vi "PLAN_CREATOR.vi"(8 "error In":errorcluster) -> (0 "error out":errorcluster)   [LabVIEW 2017]
uses:
  <vilib>/Utility/error.llb/DialogType.ctl
  Controls/Ass. Loop Control.ctl
panel:
  in  "PLAN NAME":string(combo)
  in  "CURRENT PLAN TABLE":string[][](table)
  in  "REMOVE PART":bool
  in  "ADD PART":bool
  in  "LIST OF PARTS":string(combo)
  in  "DOORS":string(combo)
  out "USER:-":string
  in  "Stop":bool
  out "DATE/TIME":string
  out "Screen Name":string
  # "Nm"
  # "NOT IN USE"
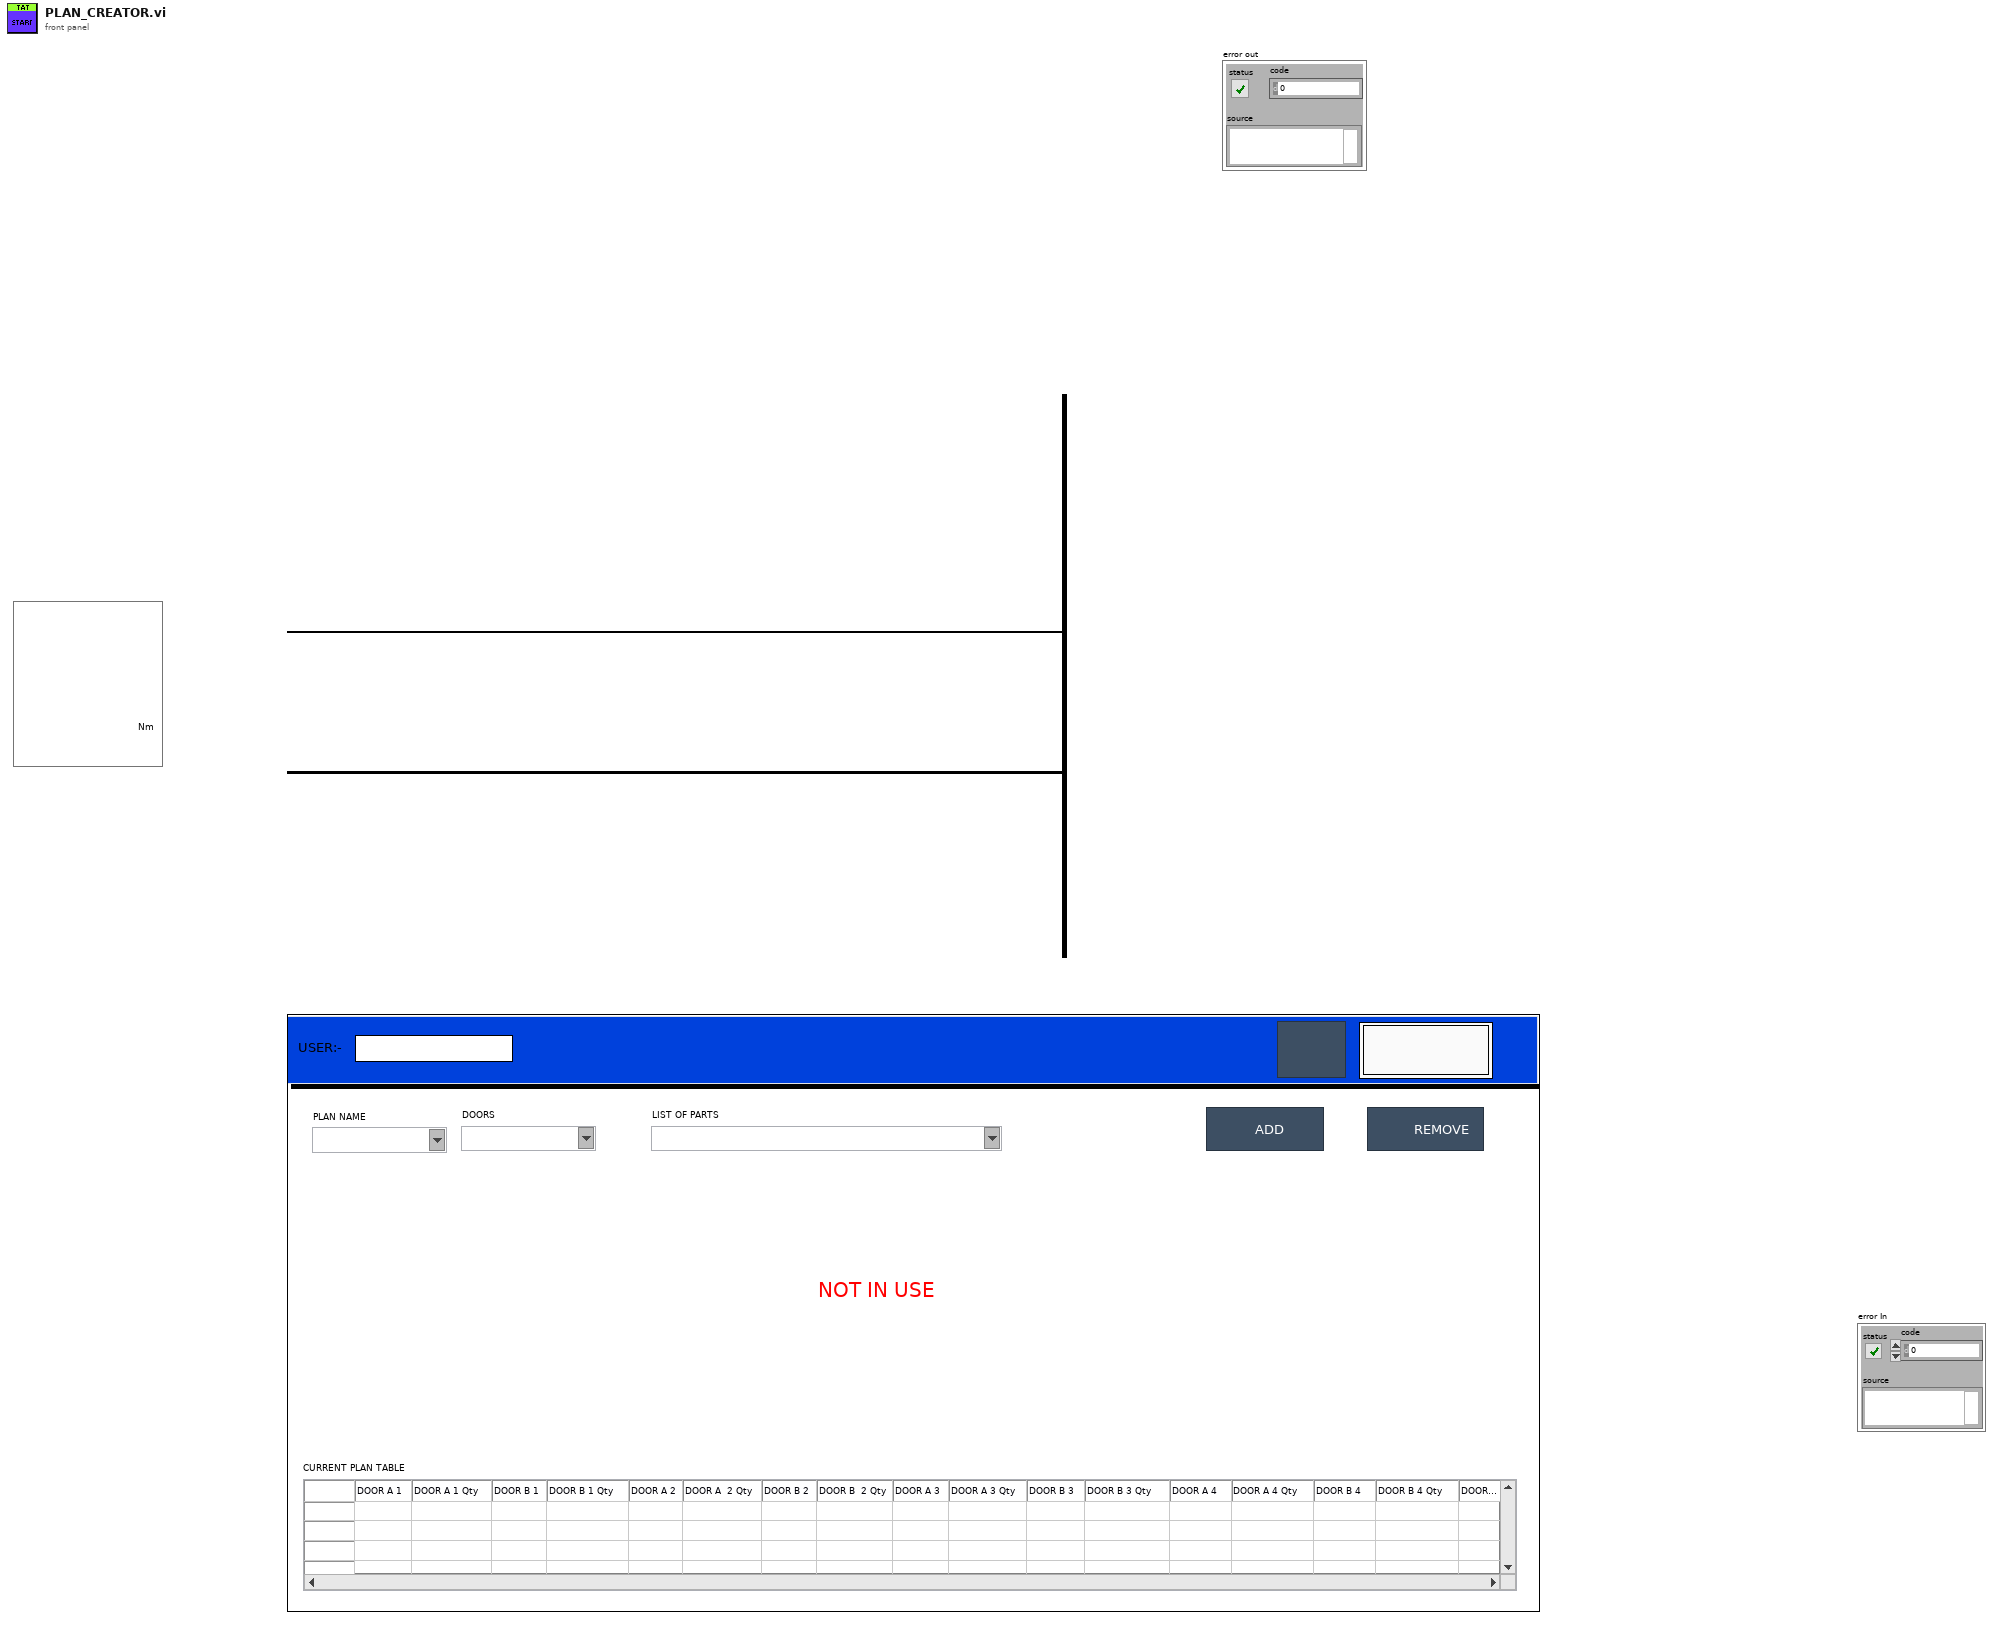
[diagram p1: front panel]
types:
  T1 = typedef "DialogType.ctl" = u16
  T2 = enum32{"invalid app kind", "Development System", "Run Time System", "Student Edition", "Embedded LabVIEW", "Evaluation", "Custom"}
  T3 = typedef "Ass. Loop Control.ctl" = enum16{"Package_Qty_Count", "GENERATE_QR_PRNT", "Cluster_update", "Waiting_for_scan", "barcode CHECK", "Int", "SaveReport ", "Barcode Print", "Start Cycle", "Wait", "Cycle End", "Stop"}
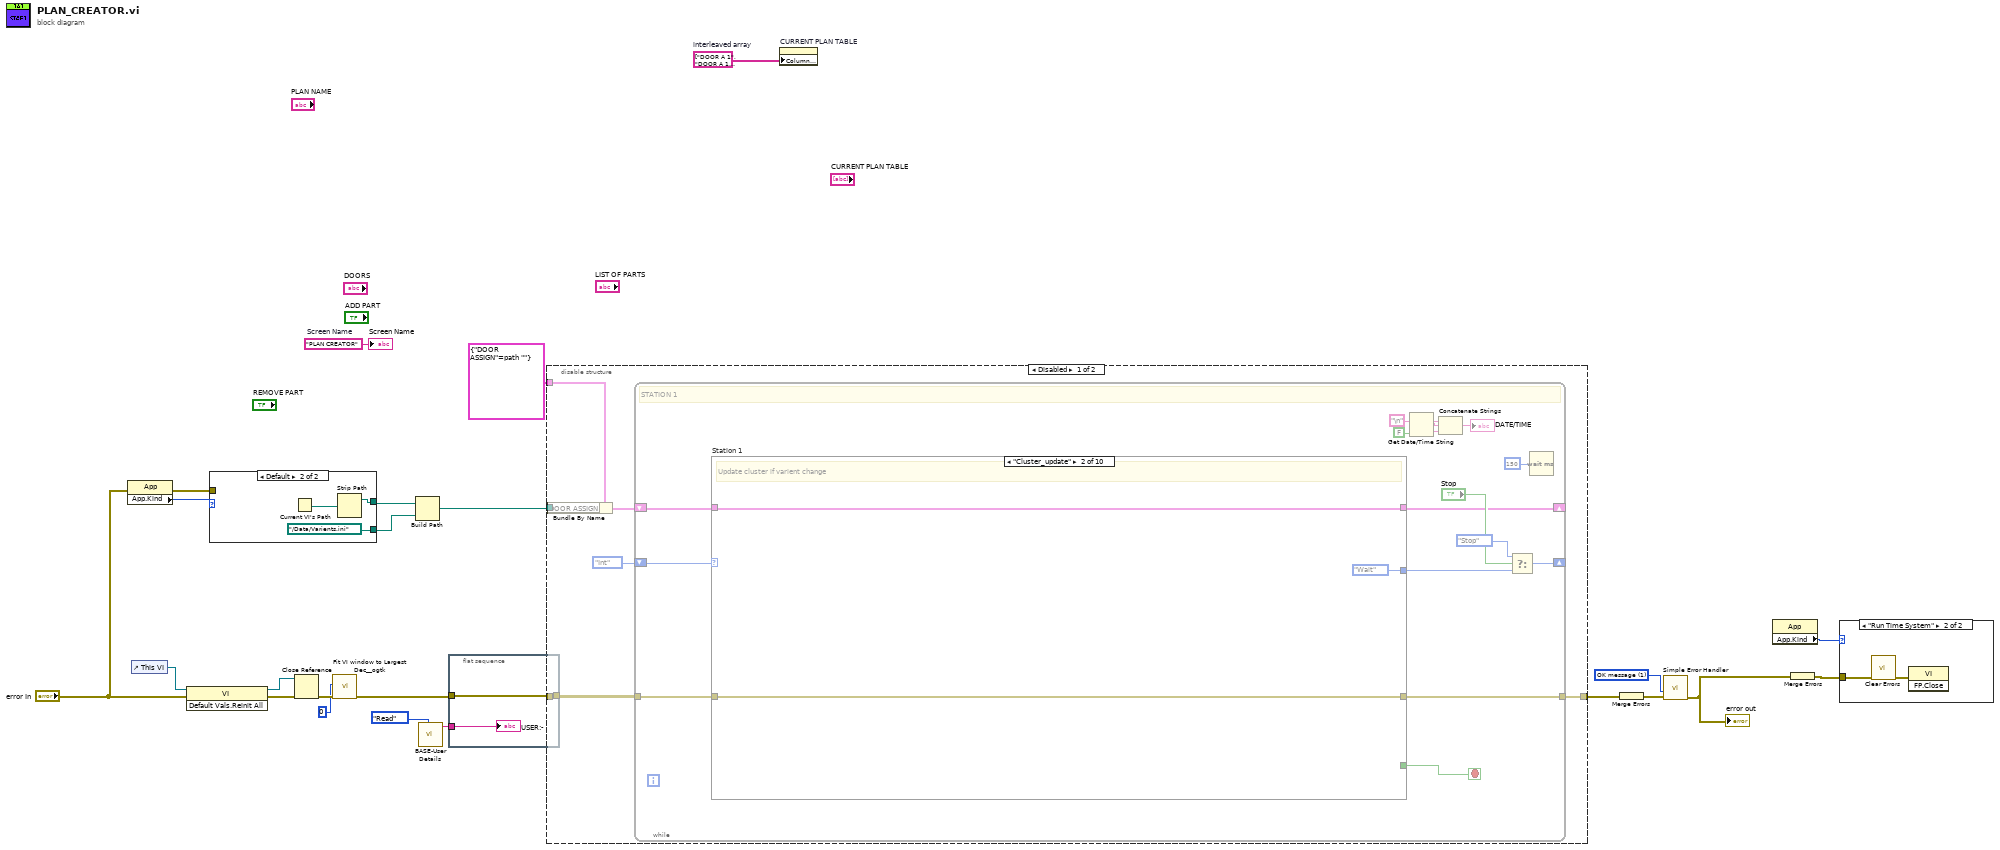
[diagram p0: block diagram]
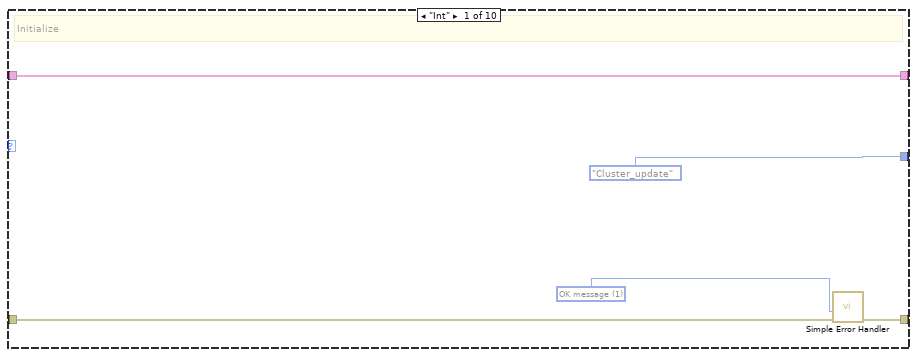
[diagram p2: hidden frame]
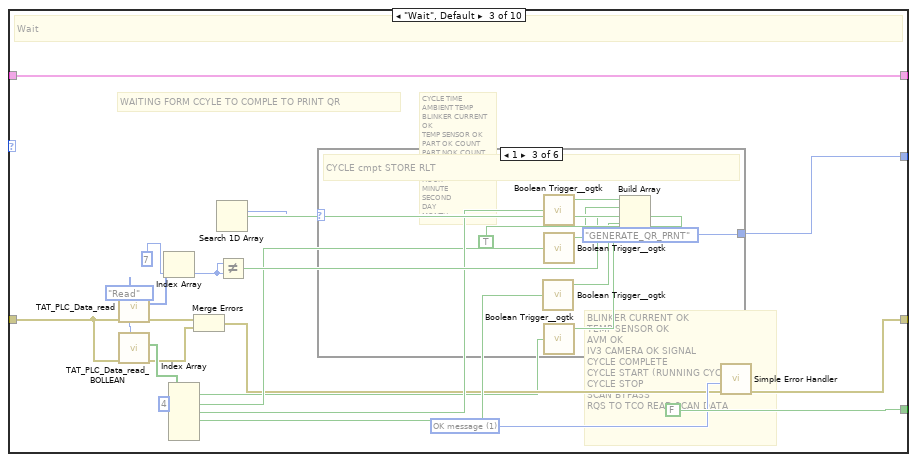
[diagram p3: hidden frame]
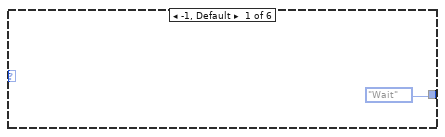
[diagram p4: hidden frame]
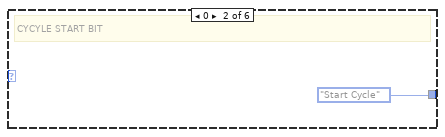
[diagram p5: hidden frame]
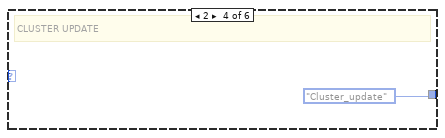
[diagram p6: hidden frame]
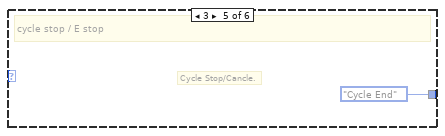
[diagram p7: hidden frame]
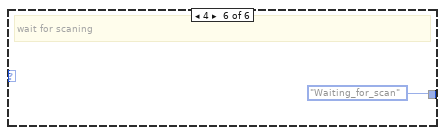
[diagram p8: hidden frame]
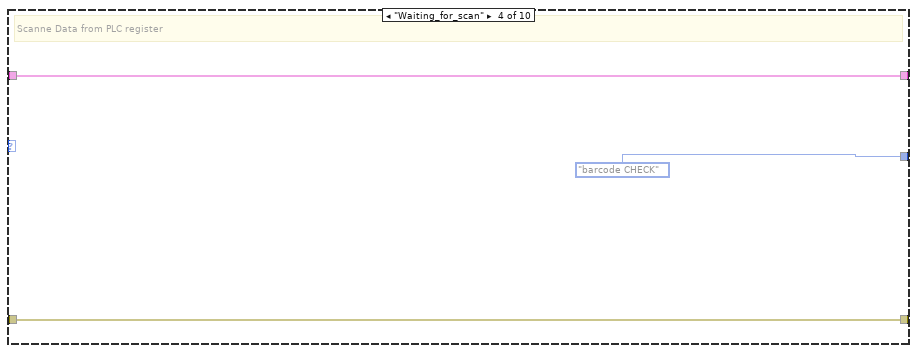
[diagram p9: hidden frame]
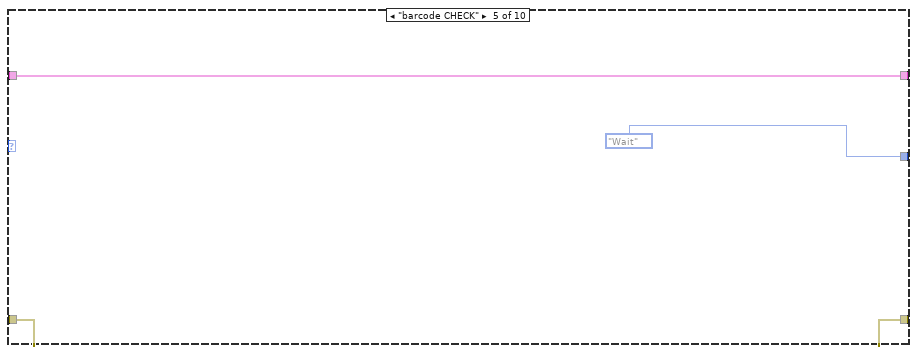
[diagram p10: hidden frame]
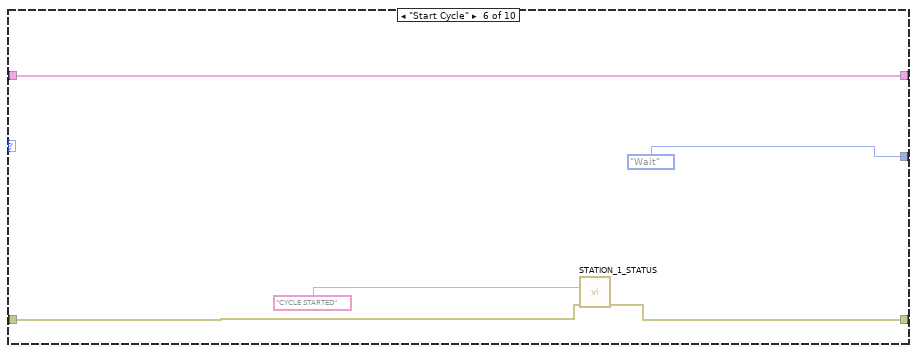
[diagram p11: hidden frame]
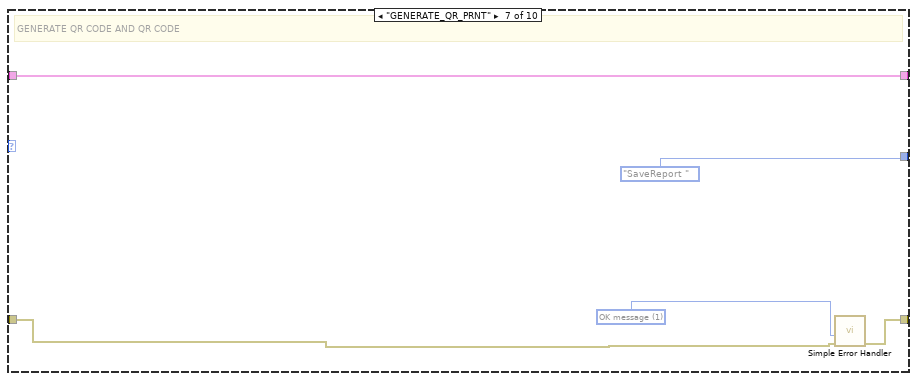
[diagram p12: hidden frame]
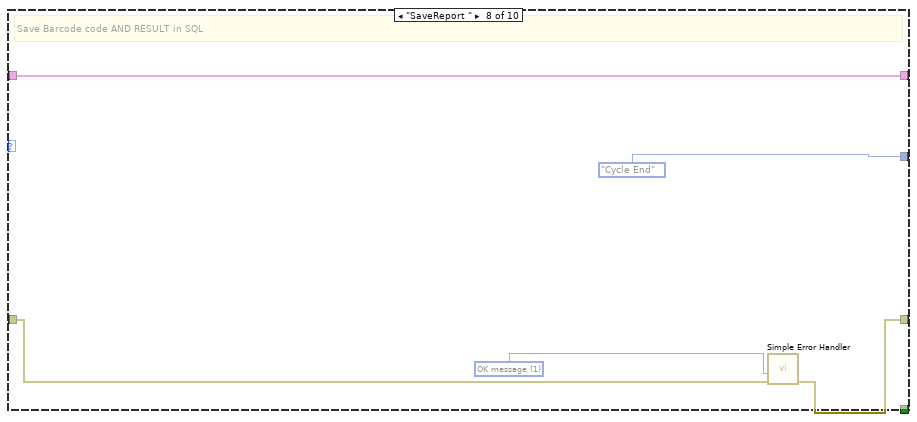
[diagram p13: hidden frame]
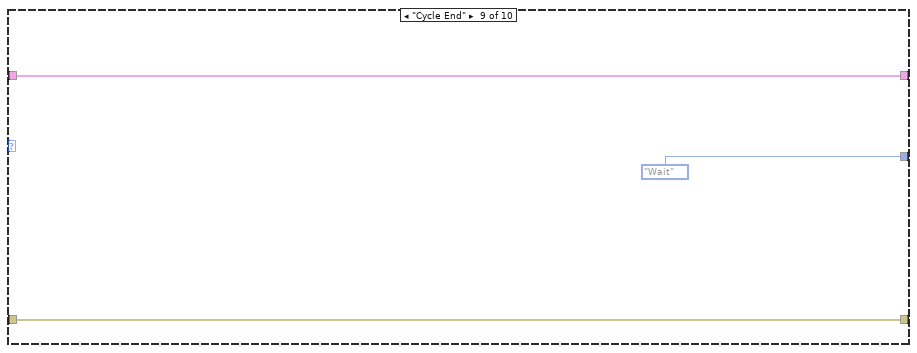
[diagram p14: hidden frame]
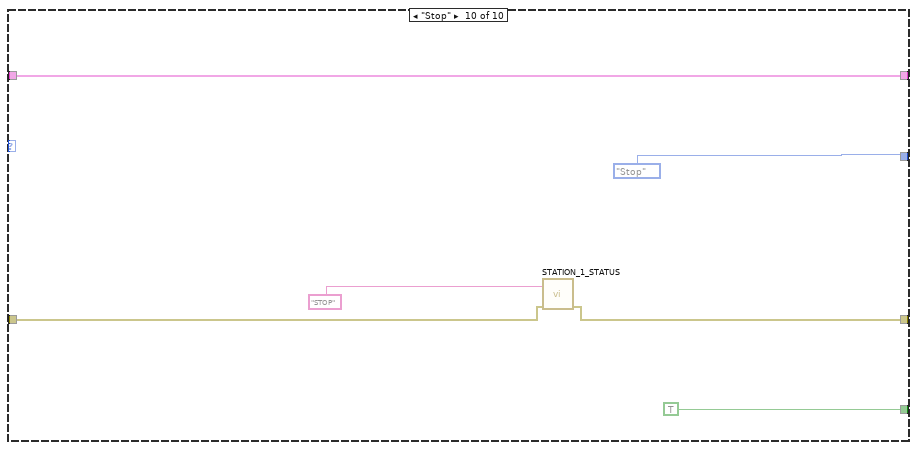
[diagram p15: hidden frame]
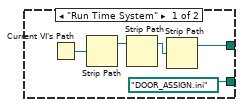
[diagram p17: hidden frame]
diagram:
  w1 = string[] ["DOOR A 1", "DOOR A 1 Qty", "DOOR B 1", "DOOR B 1 Qty", "DOOR A 2", "DOOR A  2 Qty", "DOOR B 2", "DOOR B  2 Qty", "DOOR A 3", "DOOR A 3 Qty", "DOOR B 3", "DOOR B 3 Qty", "DOOR A 4", "DOOR A 4 Qty", "DOOR B 4", "DOOR B 4 Qty", "DOOR A 5", "DOOR A 5 Qty", "DOOR B 5", "DOOR B 5 Qty", "DOOR A 11", "DOOR A 11 Qty", "DOOR B 11", "DOOR B 11 Qty", "DOOR A 12", "DOOR A 12 Qty", "DOOR B 12", "DOOR B 12 Qty", "DOOR A 13", "DOOR A 13 Qty", "DOOR B 13", "DOOR B 13 Qty", "DOOR A 14", "DOOR A 14 Qty", "DOOR B 14", "DOOR B 14 Qty", "DOOR A 15", "DOOR A 15 Qty", "DOOR B 15", "DOOR B 15 Qty", "DOOR A 16", "DOOR A 16 Qty", "DOOR B 16", "DOOR B 16 Qty"]  # interleaved array
  w4 = "PLAN CREATOR"  # Screen Name
  w16 = T1 1 items=["no dialog", "OK message", "continue or stop message", "OK message + warnings", "continue/stop + warnings"] ("type of dialog (OK msg:1)")
  n1 = property class="App"(error in="error In") -> (error out=w12:errorcluster, "App.Kind"=w14:T2)  [unwired: 1 in, 1 out]
  n2 = control-ref of="This VI"() -> (w24:refnum<vi>)
  n3 = invoke class="VI" method="Default Vals.Reinit All"(reference=w24, error in="error In") -> (reference out=w22:refnum<vi>, error out=w23:errorcluster)  [unwired: 1 in, 1 out]
  n4 = case shown="Default" w14 {
    tunnel: [path "DOOR_ASSIGN.ini" ("path") path "../Data/Varients.ini" ("path")] -> w13
    tunnel: [w25 w30] -> w6
    tunnel: w12 -> [_ _]
    frame "Run Time System" {
      n5 = Current VI's Path() -> (path=w28:path)
      n6 = Strip Path(path=w28) -> (stripped path=w27:path)  [unwired: 1 out]
      n7 = Strip Path(path=w27) -> (stripped path=w26:path)  [unwired: 1 out]
      n8 = Strip Path(path=w26) -> (stripped path=w25:path)  [unwired: 1 out]
    }
    frame Default {
      n9 = Current VI's Path() -> (path=w31:path)
      n10 = Strip Path(path=w31) -> (stripped path=w30:path)  [unwired: 1 out]
    }
  }
  n11 = Close Reference(reference=w22, error in (no error)=w23) -> (error out=w21:errorcluster)
  n12 = call <userlib>:"Fit VI window to Largest Dec__ogtk.vi"("error in (no error)"=w21, "border spacing (2 px)"=0) -> ("error out"=w10:errorcluster)  [unwired: 4 in, 1 out]
  n13 = Build Path(base path=w6, name or relative path=w13) -> (appended path=w2:path)
  n14 = call "BASE-User Details.vi"("Enum"=enum16{"Read", "Write"}."Read") -> ("User Name Out"=w17:string)  [unwired: 9 in, 1 out]
  n15 = flat-sequence {
    tunnel: [w34] -> w5
    tunnel: w10 -> [w34]
    tunnel: w17 -> [w33]
    frame #0 {
      "USER:-" <- w33
    }
  }
  n16 = disable-structure shown="Disabled" {
    disable-tunnel: [w39 _] -> w20
    disable-tunnel: w5 -> [w38 _]
    disable-tunnel: cluster{"DOOR ASSIGN":path} {"DOOR ASSIGN"=path ""} -> [w37 _]
    disable-tunnel: w2 -> [w36 _]
    frame Disabled {
      n17 = Bundle By Name(cluster=w37, "DOOR ASSIGN"=w36) -> (w35:cluster{"DOOR ASSIGN":path})
      n18 = while {
        tunnel: w38 -> [w43]
        shift-right: [w53] -> _
        shift-left: Ass._Loop_Control."Int" ("Enum") -> [w56]
        tunnel: [w54] -> w39
        shift-right: [w41] -> _
        shift-left: w35 -> [w42]
        stop <- w46 stop-if-true
        # "STATION 1"
        n19 = case "Station 1" shown="\"Cluster_update\"" w56 {
          tunnel: [Ass._Loop_Control."Cluster_update" ("Enum") Ass._Loop_Control."Wait" ("Enum") w85 Ass._Loop_Control."barcode CHECK" ("Enum") Ass._Loop_Control."Wait" ("Enum") Ass._Loop_Control."Wait" ("Enum") Ass._Loop_Control."SaveReport " ("Enum") Ass._Loop_Control."Cycle End" ("Enum") Ass._Loop_Control."Wait" ("Enum") Ass._Loop_Control."Stop" ("Enum")] -> w45
          tunnel: [_ _ FALSE _ _ _ _ _ _ TRUE] -> w46
          tunnel: [w59 w63 w82 w99 w102 w105 w112 w116 w120 w123] -> w54
          tunnel: w43 -> [w58 w63 w79 w99 w102 w106 w110 w115 w120 w124]
          tunnel: w42 -> [w57 w62 w65 w98 w101 w104 w109 w114 w119 w122]
          tunnel: [w57 w62 w65 w98 w101 w104 w109 w114 w119 w122] -> w41
          frame "Int" {
            w60 = T1 1 items=["no dialog", "OK message", "continue or stop message", "OK message + warnings", "continue/stop + warnings"] ("type of dialog (OK msg:1)")
            # "Initialize"
            n20 = call <vilib>:"Simple Error Handler.vi"("type of dialog (OK msg:1)"=w60, "error in (no error)"=w58) -> ("error out"=w59:errorcluster)  [unwired: 3 in, 4 out]
          }
          frame "Cluster_update" {
            # "Update cluster if varient change"
          }
          frame "Wait", Default {
            w83 = T1 1 items=["no dialog", "OK message", "continue or stop message", "OK message + warnings", "continue/stop + warnings"] ("type of dialog (OK msg:1)")
            w80 = enum16{"Read", "Write"}."Read" ("Enum")
            # "CYCLE TIME\nAMBIENT TEMP\nBLINKER CURRENT OK\nTEMP SENSOR OK\nPART OK COUNT\nPART NOK COUNT\nFAULT BIT\nVARIENT\nHOUR\nMINUTE\nSECOND\nDAY\nMONTH\nYEAR\nSERIAL NUMBER"
            # "BLINKER CURRENT OK\nTEMP SENSOR OK\nAVM OK\nIV3 CAMERA OK SIGNAL\nCYCLE COMPLETE\nCYCLE START (RUNNING CYCLE)\nCYCLE STOP\nSCAN BYPASS\nRQS TO TCO READ SCAN DATA"
            # "WAITING FORM CCYLE TO COMPLE TO PRINT QR"
            # "Wait"
            n21 = call "TAT_PLC_Data_read.vi"("Enum"=w80, "error in (no error)"=w79) -> ("error out"=w70:errorcluster, "Array 2"=w86:u16[])  [unwired: 8 in]
            n22 = call "TAT_PLC_Data_read_BOLLEAN.vi"("Enum"=w80, "error in (no error)"=w79) -> ("error out"=w68:errorcluster, "Array 2"=w78:bool[])  [unwired: 8 in]
            n23 = Index Array(array=w86, index=7) -> (element=w66:u16)
            n24 = Index Array(array=w78, index #1=4 ("index")) -> (element #1=w75:bool, element #2=w76:bool, element #3=w74:bool, element #5=w67:bool)  [unwired: 4 in, 1 out]
            n25 = Merge Errors(w70, w68) -> (w69:errorcluster)
            n26 = Not Equal?(x=w66, y=w66) -> (x != y?=w84:bool)
            n27 = call <userlib>:"Boolean Trigger__ogtk.vi"("Boolean Input"=w74) -> ("Rising Edge"=w73:bool)  [unwired: 1 in, 1 out]
            n28 = call <userlib>:"Boolean Trigger__ogtk.vi"("Boolean Input"=w76) -> ("Rising Edge"=w90:bool)  [unwired: 1 in, 1 out]
            n29 = call <userlib>:"Boolean Trigger__ogtk.vi"("Boolean Input"=w75) -> ("Rising Edge"=w81:bool)  [unwired: 1 in, 1 out]
            n30 = call <userlib>:"Boolean Trigger__ogtk.vi"("Boolean Input"=w67) -> ("Rising Edge"=w72:bool)  [unwired: 1 in, 1 out]
            n31 = Build Array(w90, w81, w84, w73, w72) -> (w89:bool[])
            n32 = Search 1D Array(1D array=w89, element=TRUE ("Boolean Input")) -> (index of element=w88:i32)  [unwired: 1 in]
            n33 = case shown="1" w88 {
              tunnel: [Ass._Loop_Control."Wait" ("Enum") Ass._Loop_Control."Start Cycle" ("Enum") Ass._Loop_Control."GENERATE_QR_PRNT" ("Enum") Ass._Loop_Control."Cluster_update" ("Enum") Ass._Loop_Control."Cycle End" ("Enum") Ass._Loop_Control."Waiting_for_scan" ("Enum")] -> w85
              frame -1, Default {
              }
              frame 0 {
                # "CYCYLE START BIT"
              }
              frame 1 {
                # "CYCLE cmpt STORE RLT"
              }
              frame 2 {
                # "CLUSTER UPDATE"
              }
              frame 3 {
                # "Cycle Stop/Cancle."
                # "cycle stop / E stop"
              }
              frame 4 {
                # "wait for scaning"
              }
            }
            n34 = call <vilib>:"Simple Error Handler.vi"("type of dialog (OK msg:1)"=w83, "error in (no error)"=w69) -> ("error out"=w82:errorcluster)  [unwired: 3 in, 4 out]
          }
          frame "Waiting_for_scan" {
            # "Scanne Data from PLC register"
          }
          frame "barcode CHECK" {
          }
          frame "Start Cycle" {
            n35 = call "STATION_1_STATUS.vi"("error in (no error)"=w106, "STATUS"="CYCLE STARTED" ("Cycle Status")) -> ("error out"=w105:errorcluster)  [unwired: 9 in]
          }
          frame "GENERATE_QR_PRNT" {
            w113 = T1 1 items=["no dialog", "OK message", "continue or stop message", "OK message + warnings", "continue/stop + warnings"] ("type of dialog (OK msg:1)")
            # "GENERATE QR CODE AND QR CODE"
            n36 = call <vilib>:"Simple Error Handler.vi"("type of dialog (OK msg:1)"=w113, "error in (no error)"=w110) -> ("error out"=w112:errorcluster)  [unwired: 3 in, 4 out]
          }
          frame "SaveReport " {
            w117 = T1 1 items=["no dialog", "OK message", "continue or stop message", "OK message + warnings", "continue/stop + warnings"] ("type of dialog (OK msg:1)")
            # "Save Barcode code AND RESULT in SQL"
            n37 = call <vilib>:"Simple Error Handler.vi"("type of dialog (OK msg:1)"=w117, "error in (no error)"=w115) -> ("error out"=w116:errorcluster)  [unwired: 3 in, 4 out]
          }
          frame "Cycle End" {
          }
          frame "Stop" {
            n38 = call "STATION_1_STATUS.vi"("error in (no error)"=w124, "STATUS"="STOP" ("Cycle Status")) -> ("error out"=w123:errorcluster)  [unwired: 9 in]
          }
        }
        n39 = Get Date/Time String(want seconds? (F)=FALSE) -> (date string=w50:string, time string=w49:string)  [unwired: 2 in]
        n40 = Concatenate Strings(w50, "\n", w49) -> (→"DATE/TIME":string)
        n41 = Select(t=Ass._Loop_Control."Stop" ("Enum"), s="Stop", f=w45) -> (s? t:f=w53:T3)
        n42 = Wait (ms)(milliseconds to wait=u32 150) -> ()  [unwired: 1 out]
      }
    }
    frame Enabled {
    }
  }
  n43 = property on="CURRENT PLAN TABLE" class="Tbl (strict)"("Column Headers[]"=w1) -> ()  [unwired: 2 in, 2 out]
  n44 = Merge Errors(w20) -> (w19:errorcluster)
  n45 = call <vilib>:"Simple Error Handler.vi"("type of dialog (OK msg:1)"=w16, "error in (no error)"=w19) -> ("error out"=w7:errorcluster)  [unwired: 3 in, 4 out]
  "error out" <- w7
  n46 = property class="App"() -> ("App.Kind"=w15:T2)  [unwired: 2 in, 2 out]
  n47 = Merge Errors(w7) -> (w8:errorcluster)
  n48 = case shown="\"Run Time System\"" w15 {
    tunnel: w8 -> [_ w129]
    frame "invalid app kind", Default {
    }
    frame "Run Time System" {
      n49 = call <vilib>:"Clear Errors.vi"("error in (no error)"=w129) -> ("error out"=w128:errorcluster)  [unwired: 5 in, 1 out]
      n50 = invoke class="VI" method="FP.Close"(error in=w128) -> ()  [unwired: 2 in, 3 out]
    }
  }
  "Screen Name" <- w4
